vi "get default error list.vi"(8 "error in (no error)":errorcluster, 11 "fixed channel configuration in":refnum<class "user control module configuration.lvclass">) -> (0 "error out":errorcluster, 2 "error list":T1[](array[typedef]), 3 "fixed channel configuration out":refnum<class "user control module configuration.lvclass">)   [LabVIEW 2013, in "user control module configuration.lvclass"]
uses:
  user control module configuration.lvclass
  <vilib>/NI/Tag Bus Module Framework/runtime/error classification.ctl
  <vilib>/NI/Tag Bus Module Framework/runtime/TBM module execution interface.lvclass
  <vilib>/NI/DCAF/Tag Editor Core/control module/configuration/error classification setting.ctl
  <vilib>/NI/DCAF/Tag Editor Core/control module/configuration/control module configuration.lvclass
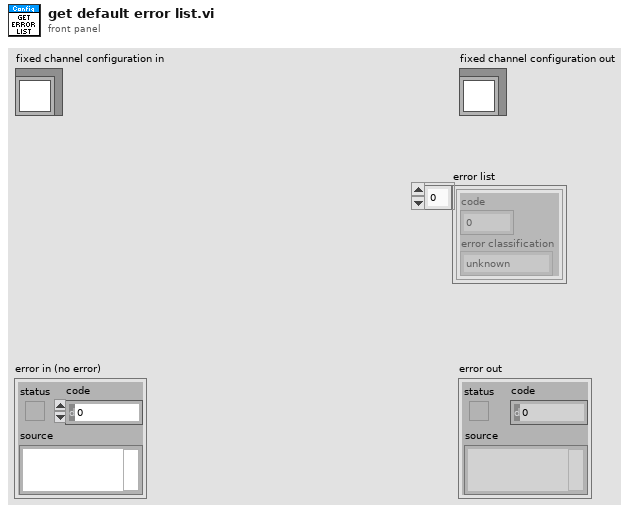
[diagram p1: front panel]
types:
  T1 = typedef "control module configuration.lvclass/error classification setting.ctl" = cluster{"code":i32, "error classification":T2}
  T2 = typedef "TBM module execution interface.lvclass/error classification.ctl" = enum16{"unknown", "none", "trivial", "recoverable", "critical"}
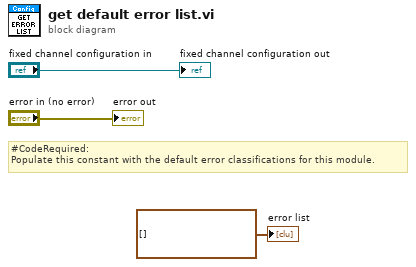
[diagram p0: block diagram]
diagram:
  # "#CodeRequired:\nPopulate this constant with the default error classifications for this module."
  "error out" <- "error in (no error)"
  "fixed channel configuration out" <- "fixed channel configuration in"
  "error list" <- T1[] [] ("error list")
